vi "PRIVATE.ProcCases.vi"(0 "i ref in":refnum<vi>, 1 "selector":string, 2 "Data":string, 3 "call cluster":T1={"Object"="", "Selector"="", "CallType"=enum."synchronous", "Async Object"="", "Async Selector"="", "Data Descriptor"="", "Data"=[], "Error #"=0, "Expire"=0}, 5 "error in (no error)":errorcluster) -> (14 "i ref out":refnum<vi>, 17 "answer cluster":T1={"Object"="", "Selector"="", "CallType"=enum."synchronous", "Async Object"="", "Async Selector"="", "Data Descriptor"="", "Data"=[], "Error #"=0, "Expire"=0}, 19 "error out":errorcluster)   [LabVIEW 2009]
doc: "This method is called by a process from within the default case in the event loop. The methods of a class that are linked to events will be called from THIS method. Add your code here."
uses:
  CSCore/CSSystem/CoreDefs/CoreDefs.call_type.ctl
  CSCore/CSSystem/CoreDefs/CoreDefs.rawDataType.ctl
  CSCore/BaseProcess/BaseProcess.descriptor string definition.ctl
  CSCore/BaseProcess/BaseProcess.lvlib
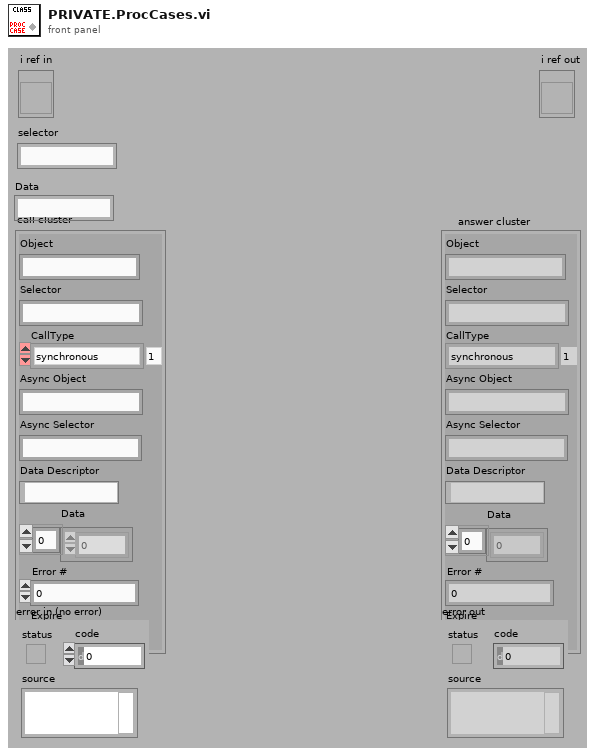
[diagram p1: front panel]
types:
  T1 = typedef "CoreDefs.call_type.ctl" = cluster{"Object":string, "Selector":string, "CallType":enum16{"simple", "synchronous", "asynchronous"}, "Async Object":string, "Async Selector":string, "Data Descriptor":T2, "Data":T3, "Error #":i32, "Expire":u32}
  T2 = typedef "BaseProcess.lvlib/BaseProcess.descriptor string definition.ctl" = string
  T3 = typedef "CoreDefs.rawDataType.ctl" = i8[]
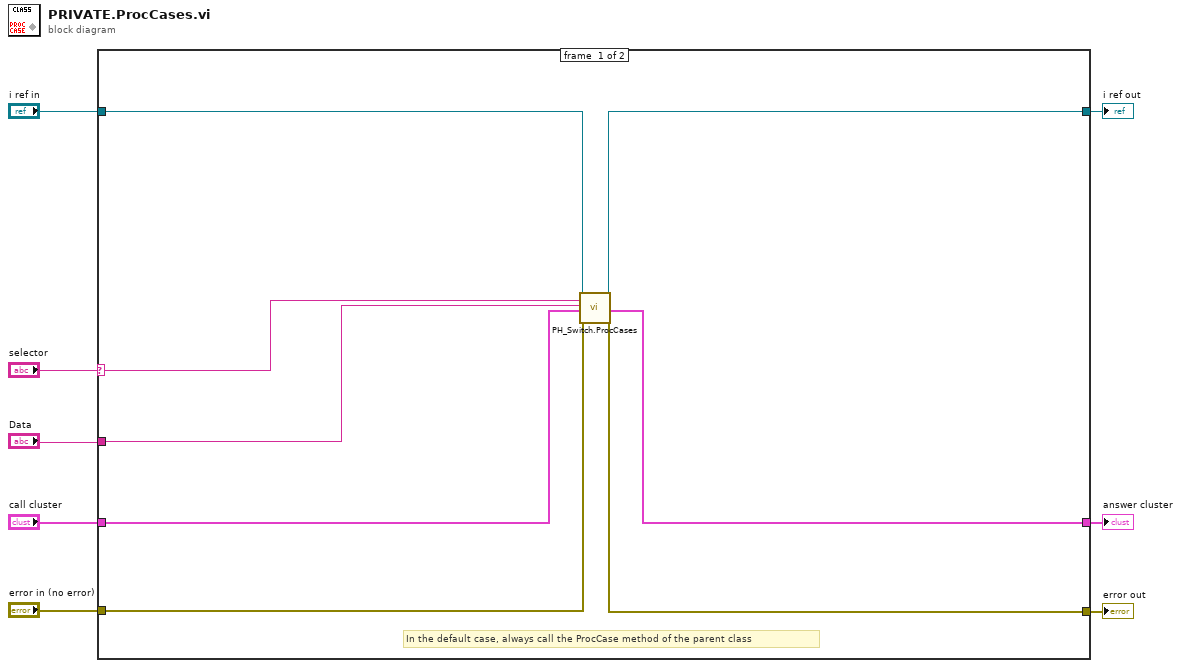
[diagram p0: block diagram]
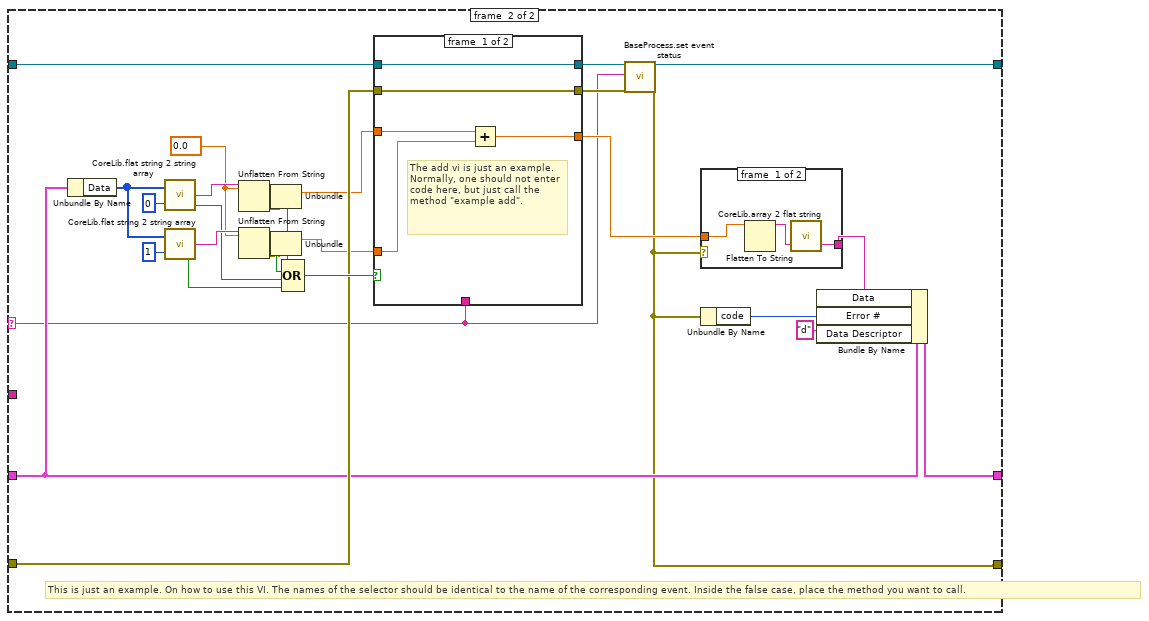
[diagram p2: hidden frame]
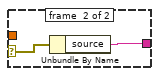
[diagram p3: hidden frame]
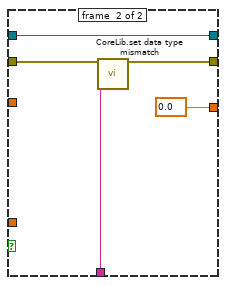
[diagram p4: hidden frame]
diagram:
  n1 = case shown="Default" "selector" {
    selector: "selector" -> [w10 w22]
    tunnel: "Data" -> [w11 _]
    tunnel: "i ref in" -> [w9 w33]
    tunnel: [w16 w20] -> w3
    tunnel: "call cluster" -> [w12 w28]
    tunnel: [w13 w27] -> w7
    tunnel: "error in (no error)" -> [w15 w32]
    tunnel: [w14 w23] -> w1
    frame #0 {
      # "In the default case, always call the ProcCase method of the parent class"
      n2 = call "PH_Switch.ProcCases.vi"("i ref in"=w9, "selector"=w10, "Data"=w11, "call cluster"=w12, "error in (no error)"=w15) -> ("i ref out"=w16:refnum<vi>, "answer cluster"=w13:T1, "error out"=w14:errorcluster)  [unwired: 12 in]
    }
    frame #1 {
      w39 = 0.0
      # "This is just an example. On how to use this VI. The names of the selector should be identical to the name of the corresponding event. Inside the false case, place the method you want to call."
      n3 = Unbundle By Name(w28) -> ("Data"=w44:T3)
      n4 = call "CoreLib.flat string 2 string array.vi"("flattened string"=w44, "Index"=0) -> ("string element"=w41:string, "err"=w36:bool)  [unwired: 1 out]
      n5 = call "CoreLib.flat string 2 string array.vi"("flattened string"=w44, "Index"=1) -> ("string element"=w40:string, "err"=w35:bool)  [unwired: 1 out]
      n6 = Unflatten From String(type=w39, binary string=w41) -> (value=w21:dbl, error out=w17:errorcluster)  [unwired: 3 in, 1 out]
      n7 = Unflatten From String(type=w39, binary string=w40) -> (value=w31:dbl, error out=w18:errorcluster)  [unwired: 3 in, 1 out]
      n8 = Unbundle(w17) -> ("status"=w38:bool)  [unwired: 2 out]
      n9 = Unbundle(w18) -> ("status"=w37:bool)  [unwired: 2 out]
      n10 = Compound Arithmetic op=OR(w38, w37, w36, w35) -> (w34:bool)
      n11 = case shown="False" w34 {
        tunnel: [w51 w59] -> w25
        tunnel: w33 -> [w51 w59]
        tunnel: w32 -> [w52 w58]
        tunnel: [w52 w57] -> w24
        tunnel: w31 -> [w54 _]
        tunnel: [w53 0.0] -> w30
        tunnel: w22 -> [_ w55]
        tunnel: w21 -> [w50 _]
        frame #0 {
          # "The add vi is just an example. Normally, one should not enter code here, but just call the method \"example add\"."
          n12 = Add(x=w50, y=w54) -> (x+y=w53:dbl)
        }
        frame #1 {
          n13 = call "CoreLib.set data type mismatch.vi"("error in (no error)"=w58, "error source"=w55) -> ("error out"=w57:errorcluster)  [unwired: 17 in]
        }
      }
      n14 = call "BaseProcess.set event status.vi"("i ref in"=w25, "EventStatus"=w22, "error in (no error)"=w24) -> ("i ref out"=w20:refnum<vi>, "error out"=w23:errorcluster)  [unwired: 14 in, 1 out]
      n15 = case shown="No Error" w23 {
        selector: w23 -> [_ w49]
        tunnel: [w47 w48] -> w26
        tunnel: w30 -> [w45 _]
        frame #0 {
          n16 = Flatten To String(anything=w45) -> (data string=w46:string)  [unwired: 3 in, 2 out]
          n17 = call "CoreLib.array 2 flat string.vi"("flattened string"=w46) -> ("flattened string array"=w47:string)  [unwired: 1 in, 1 out]
        }
        frame #1 {
          n18 = Unbundle By Name(w49) -> ("source"=w48:string)
        }
      }
      n19 = Unbundle By Name(w23) -> ("code"=w29:i32)
      n20 = Bundle By Name(cluster=w28, "Data"=w26, "Error #"=w29, "Data Descriptor"="d") -> (w27:T1)
    }
  }
  "answer cluster" <- w7
  "i ref out" <- w3
  "error out" <- w1
